vi "Function.vi"(8 "error in (no error)":errorcluster, 10 "Numeric":i16, 11 "Two Terminal in":refnum<class "Less 0_I16.lvclass">) -> (0 "error out":errorcluster, 2 "Result":bool, 3 "Two Terminal out":refnum<class "Less 0_I16.lvclass">)   [LabVIEW 2021, in "Less 0_I16.lvclass"]
uses:
  Less 0_I16.lvclass
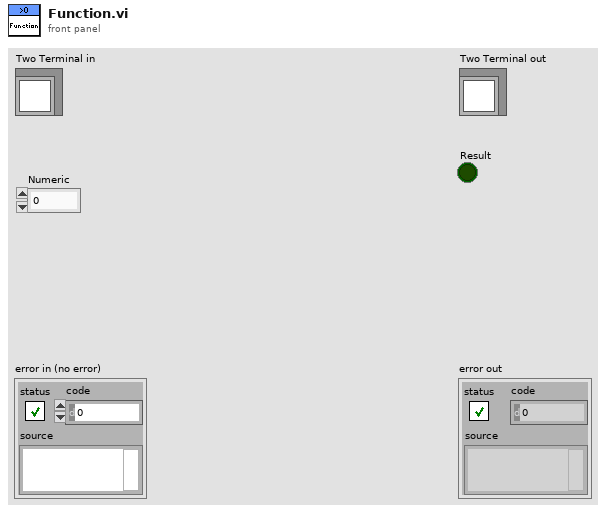
[diagram p1: front panel]
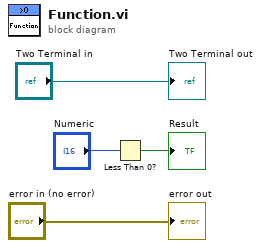
[diagram p0: block diagram]
diagram:
  n1 = Less Than 0?(x="Numeric") -> (x < 0?=→"Result":bool)
  "error out" <- "error in (no error)"
  "Two Terminal out" <- "Two Terminal in"
